vi "ManageAreaScanRoutines.vi"(0 "System no.":i32=1 min=1 step=1, 5 "error in (no error)":errorcluster) -> (19 "error out":errorcluster)   [LabVIEW 2020]
doc: "This VI allows to add or edit Area Scan Routines (FDR).\n\nRoutines can be managed on the controller directly or via text files."
uses:
  Message Cluster.ctl
  <vilib>/Utility/miscctls.llb/LVRowAndColumnTypeDef.ctl
panel:
  in  "Update from selected":bool
  in  "Calculate Velocity":bool
  in  "Mid. pos. step axis":dbl=0.1 format="%.4f"
  in  "Range step axis":dbl=0.1 format="%.4f"
  in  "Mid. pos. scan axis":dbl=0.1 format="%.4f"
  in  "Range scan axis":dbl=0.1 format="%.4f"
  in  "Name":string
  in  "Send to controller":bool
  in  "Board":i32 min=1 max=5 step=1
  in  "Threshold Level":dbl format="%.3f"
  in  "Centroid Method":i32
  in  "Target type":i32
  in  "Stop pos. option":i32
  in  "Velocity":dbl format="%.4f"
  in  "Frequency":dbl format="%.3f"
  in  "Max. rel. input level":dbl format="%.4f"
  in  "Min. rel. input level":dbl format="%.4f"
  in  "Step axis":string
  in  "Scan axis":string
  in  "stop":bool
  in  "Available Routines":string[][](table)
  # "Routine definition"
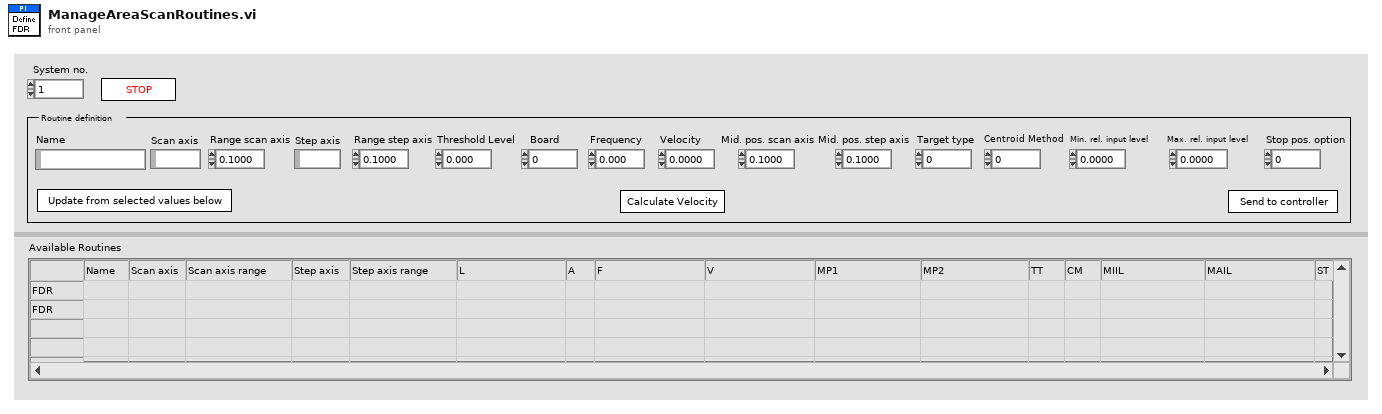
[diagram p1: front panel]
types:
  T1 = typedef "Message Cluster.ctl" = cluster{"Message":string, "Message Data":variant}
  T2 = typedef "LVRowAndColumnTypeDef.ctl" = cluster{"Row":i32, "Column":i32}
  T3 = cluster{"Scan axis":string, "Range scan axis":dbl, bool, "Mid. pos. scan axis":dbl}
  T4 = cluster{"Step axis":string, "Range step axis":dbl, bool, "Mid. pos. step axis":dbl}
  T5 = enum32{"Bad", "Idle", "Run top level", "Running"}
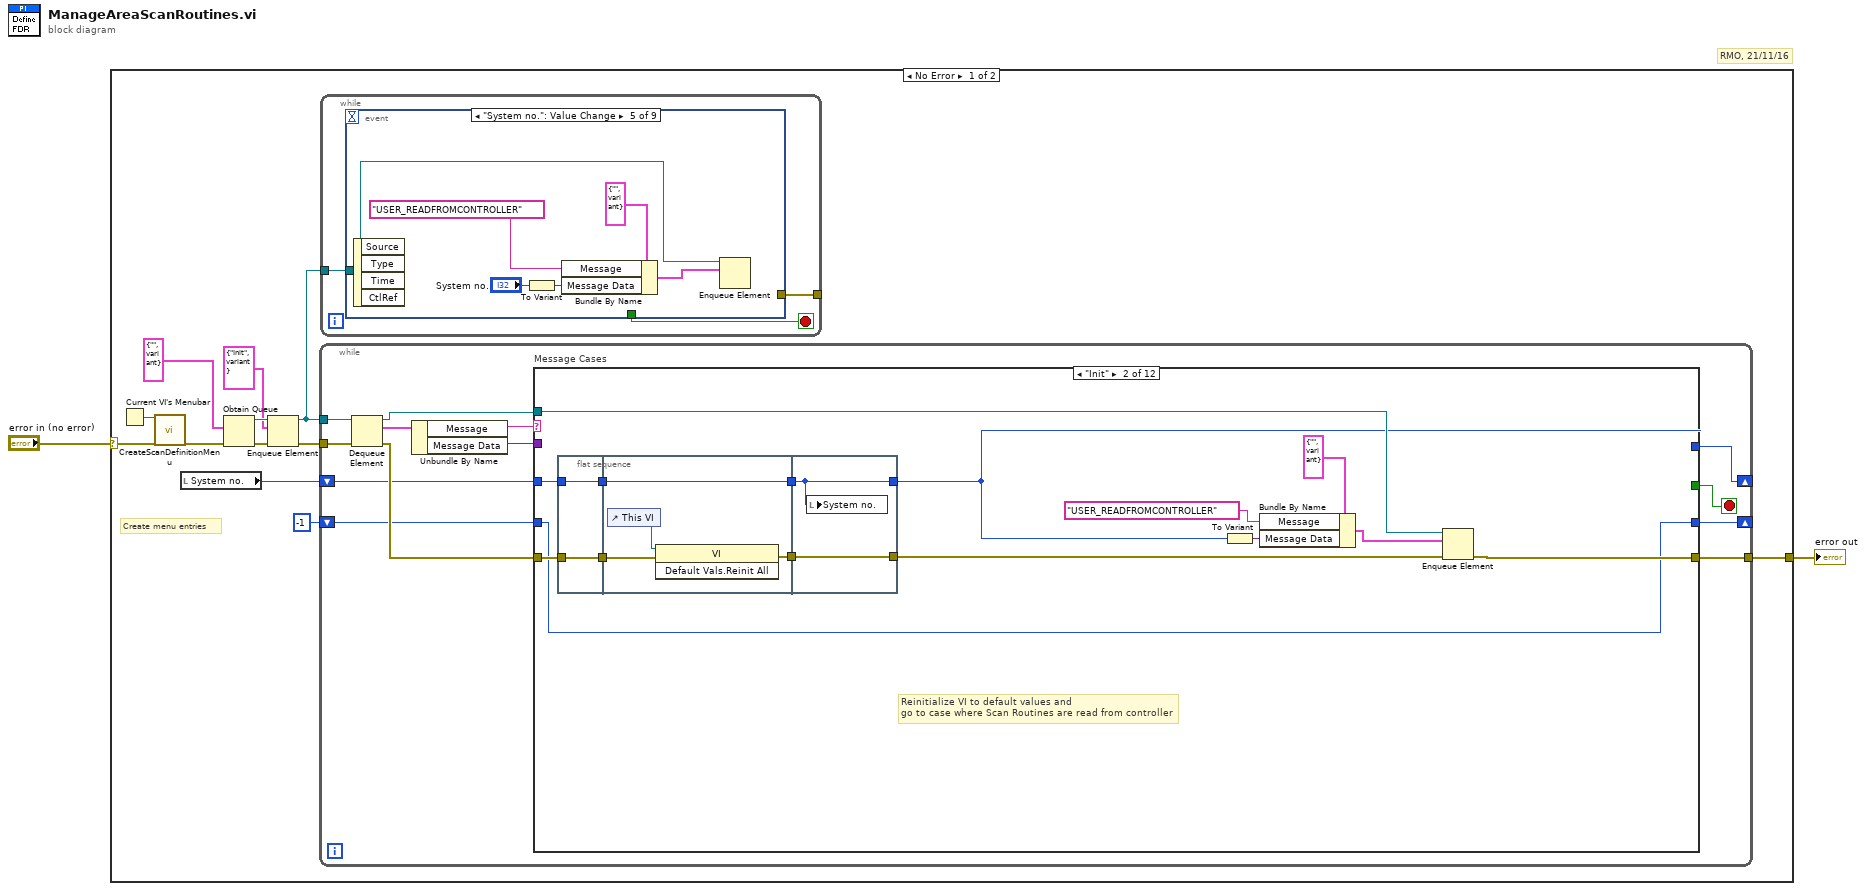
[diagram p0: block diagram]
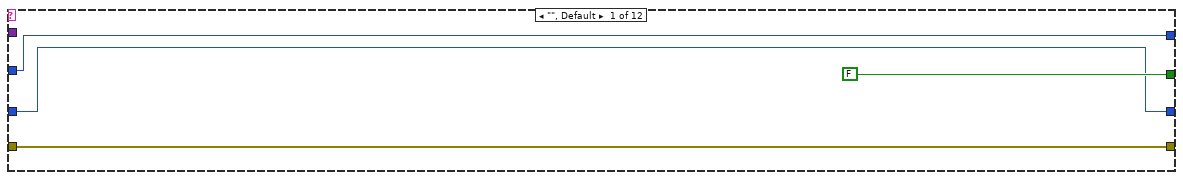
[diagram p2: hidden frame]
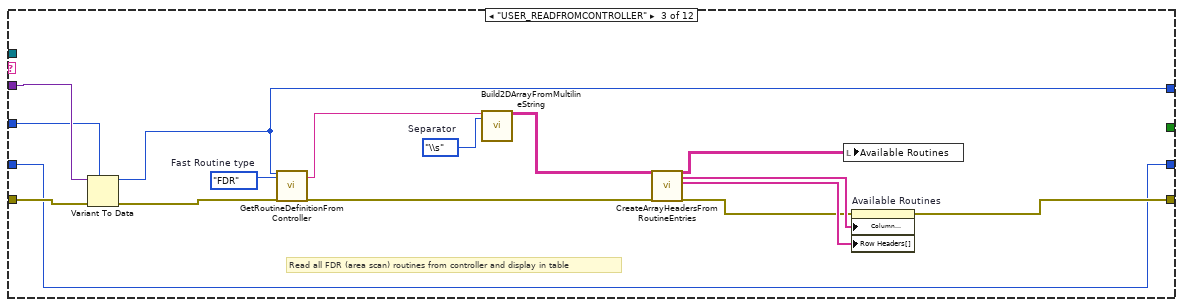
[diagram p3: hidden frame]
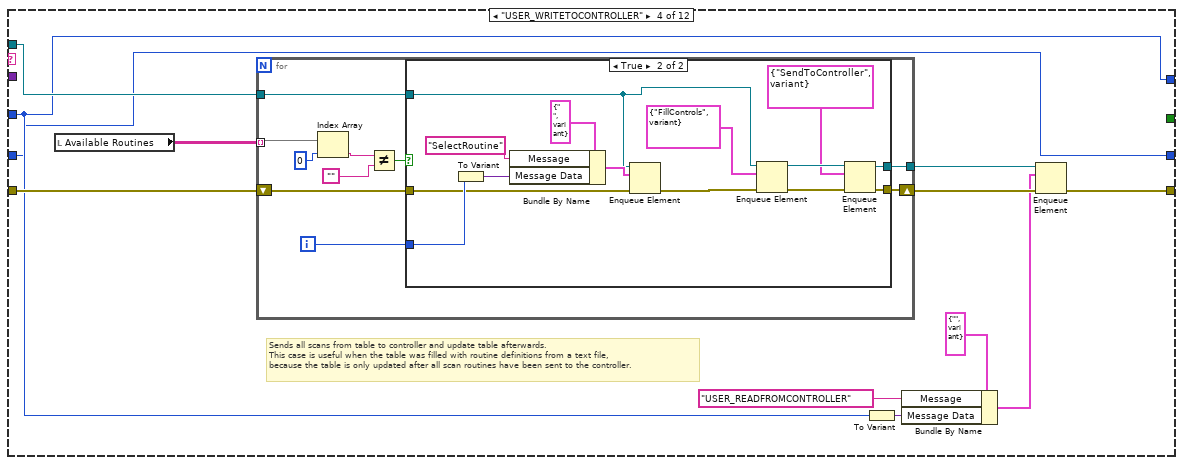
[diagram p4: hidden frame]
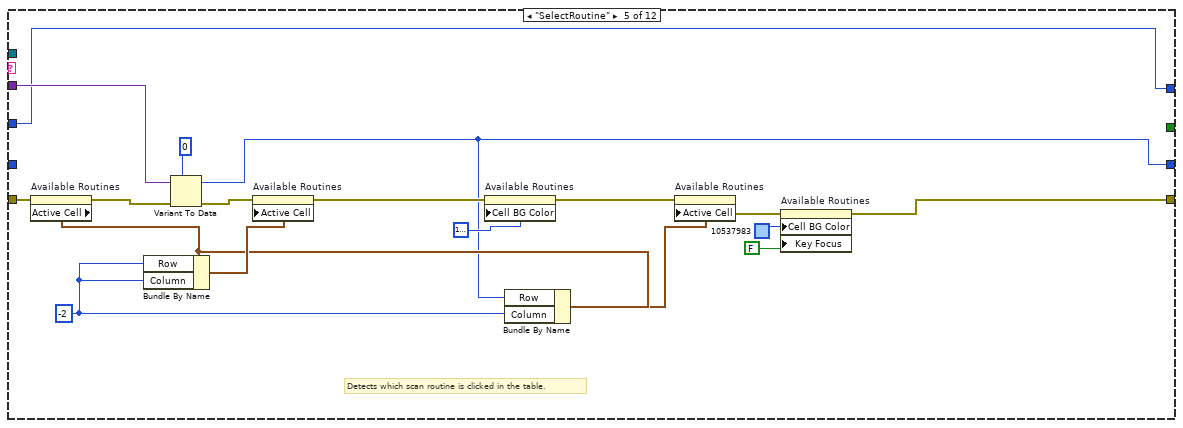
[diagram p6: hidden frame]
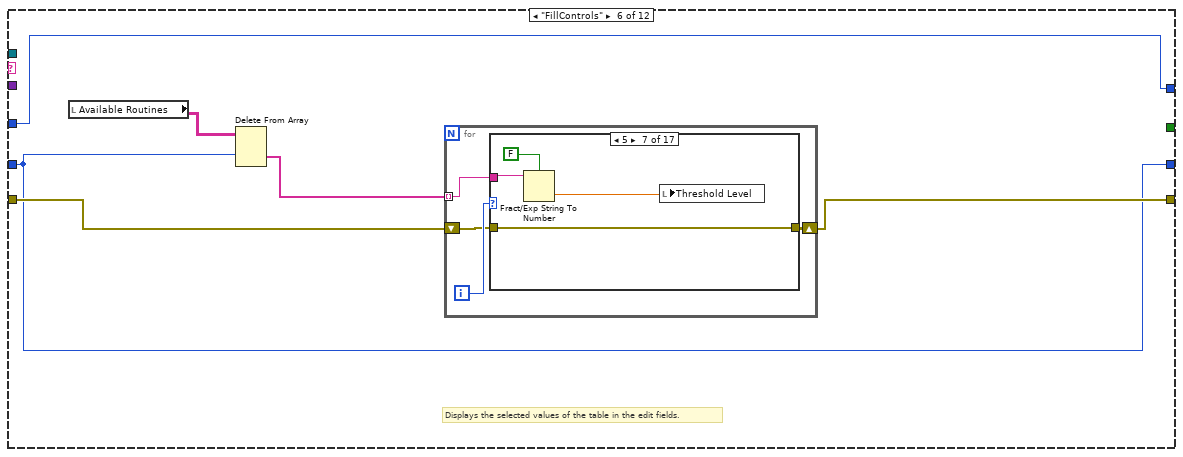
[diagram p7: hidden frame]
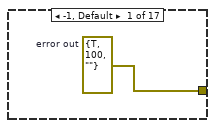
[diagram p8: hidden frame]
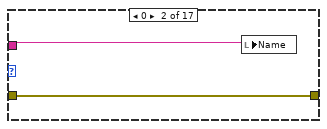
[diagram p9: hidden frame]
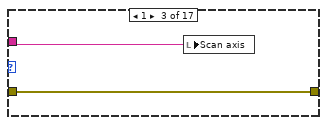
[diagram p10: hidden frame]
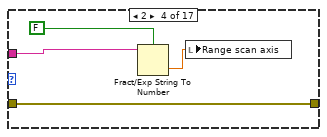
[diagram p11: hidden frame]
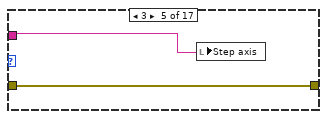
[diagram p12: hidden frame]
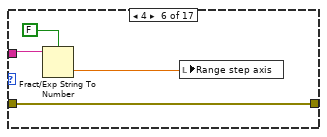
[diagram p13: hidden frame]
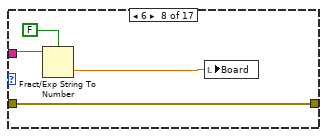
[diagram p14: hidden frame]
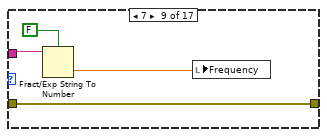
[diagram p15: hidden frame]
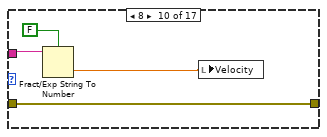
[diagram p16: hidden frame]
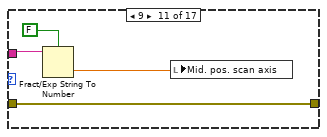
[diagram p17: hidden frame]
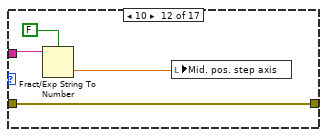
[diagram p18: hidden frame]
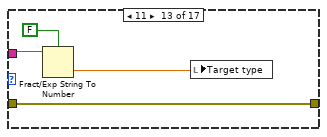
[diagram p19: hidden frame]
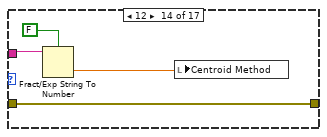
[diagram p20: hidden frame]
diagram:
  # "RMO, 21/11/16"
  n1 = case shown="No Error" "error in (no error)" {
    selector: "error in (no error)" -> [w5 w409]
    tunnel: [w6 w409] -> w2
    frame No Error {
      # "Create menu entries"
      n2 = Current VI's Menubar() -> (w14:refnum<k9>)
      n3 = call "CreateScanDefinitionMenu.vi"("menu reference"=w14, "error in (no error)"=w5) -> ("error out"=w8:errorcluster)  [unwired: 17 out]
      n4 = local read "System no."() -> (w3:i32)
      n5 = Obtain Queue(element data type=T1 {"Message"="", "Message Data"=variant} ("Message Cluster"), error in (no error)=w8) -> (queue out=w11:refnum<queue>, error out=w12:errorcluster)  [unwired: 2 in, 2 out]
      n6 = Enqueue Element(queue=w11, element=T1 {"Message"="Init", "Message Data"=variant}, error in (no error)=w12) -> (queue out=w7:refnum<queue>, error out=w9:errorcluster)  [unwired: 2 out]
      n7 = while {
        tunnel: w9 -> [w27]
        tunnel: w7 -> [w26]
        tunnel: [w21] -> w6
        shift-right: [w17] -> _
        shift-left: w3 -> [w20]
        shift-right: [w16] -> _
        shift-left: -1 ("Horizontal") -> [w15]
        stop <- w22 stop-if-true
        n8 = Dequeue Element(queue=w26, error in (no error)=w27) -> (queue out=w18:refnum<queue>, element=w25:T1, error out=w24:errorcluster)  [unwired: 2 out]
        n9 = Unbundle By Name(w25) -> ("Message"=w23:string, "Message Data"=w19:variant)
        n10 = case "Message Cases" shown="\"Init\"" w23 {
          tunnel: w24 -> [w31 w44 w61 w80 w124 w128 w203 w247 w284 w304 w331 w350]
          tunnel: [w31 w45 w64 w78 w110 w130 w202 w246 w281 w289 w333 w340] -> w21
          tunnel: [FALSE _ _ _ _ _ _ _ _ _ _ TRUE] -> w22
          tunnel: w20 -> [w29 w36 w58 w72 w111 w129 w197 w242 w280 w300 w329 w347]
          tunnel: w19 -> [_ _ w59 _ w126 _ _ _ _ _ _ _]
          tunnel: w18 -> [_ w46 _ w81 _ _ w201 _ _ _ _ _]
          tunnel: [w29 w32 w57 w72 w111 w129 w197 w242 w280 w300 w329 w347] -> w17
          tunnel: [w28 w38 w55 w71 w109 w127 w196 w241 w279 w286 w327 w339] -> w16
          tunnel: w15 -> [w28 w38 w55 w71 _ w127 w196 w241 w279 w286 w327 w339]
          frame "", Default {
          }
          frame "Init" {
            # "Reinitialize VI to default values and\ngo to case where Scan Routines are read from controller"
            n11 = flat-sequence {
              tunnel: w44 -> [w48]
              tunnel: [w48] -> w37
              tunnel: w36 -> [w47]
              tunnel: [w47] -> w35
              tunnel: w37 -> [w51]
              tunnel: w35 -> [w49]
              tunnel: [w50] -> w34
              tunnel: [w49] -> w33
              tunnel: [w54] -> w43
              tunnel: w34 -> [w54]
              tunnel: w33 -> [w53]
              tunnel: [w53] -> w32
              frame #0 {
              }
              frame #1 {
                n12 = control-ref of="This VI"() -> (w52:refnum<vi>)
                n13 = invoke class="VI" method="Default Vals.Reinit All"(reference=w52, error in=w51) -> (error out=w50:errorcluster)  [unwired: 1 in, 2 out]
              }
              frame #2 {
                n14 = local write "System no."(w53) -> ()
              }
            }
            n15 = To Variant(anything=w32) -> (Variant=w42:variant)
            n16 = Bundle By Name(cluster=T1 {"Message"="", "Message Data"=variant} ("Message Cluster"), "Message"="USER_READFROMCONTROLLER", "Message Data"=w42) -> (w40:T1)
            n17 = Enqueue Element(queue=w46, element=w40, error in (no error)=w43) -> (error out=w45:errorcluster)  [unwired: 3 out]
          }
          frame "USER_READFROMCONTROLLER" {
            w69 = enum16{"\\s", "\\t"}."\\s"  # Separator
            w70 = enum16{"FDG", "FDR"}."FDR"  # Fast Routine type
            # "Read all FDR (area scan) routines from controller and display in table"
            n18 = Variant To Data(error in=w61, type=w58, Variant=w59) -> (data=w57:i32, error out=w60:errorcluster)
            n19 = call "GetRoutineDefinitionFromController.vi"("System no."=w57, "Fast Routine type"=w70, "error in"=w60) -> ("Routine Definitons"=w56:string, "error out"=w63:errorcluster)  [unwired: 15 out]
            n20 = call "Build2DArrayFromMultilineString.vi"("String"=w56, "Separator"=w69) -> ("2D Array out"=w68:string[][])  [unwired: 17 out]
            n21 = call "CreateArrayHeadersFromRoutineEntries.vi"("Available Routines"=w68, "error in"=w63) -> ("Available Routines out"=w67:string[][], "Column Headers"=w66:string[], "Row Headers"=w65:string[], "error out"=w62:errorcluster)  [unwired: 14 out]
            n22 = local write "Available Routines"(w67) -> ()
            n23 = property on="Available Routines" class="Tbl (strict)"(error in=w62, "Column Headers[]"=w66, "Row Headers[]"=w65) -> (error out=w64:errorcluster)  [unwired: 1 in, 1 out]
          }
          frame "USER_WRITETOCONTROLLER" {
            # "Sends all scans from table to controller and update table afterwards.\nThis case is useful when the table was filled with routine definitions from a text file,\nbecause the table is only updated after all scan routines have been sent to the controller."
            n24 = local read "Available Routines"() -> (w82:string[][])
            n25 = for {
              tunnel: w82 -> [w88] mode=indexing
              tunnel: w81 -> [w91]
              shift-right: [w89] -> w79
              shift-left: w80 -> [w90]
              tunnel: [w83] -> w77
              i -> [w92]
              n26 = Index Array(array=w88, index=0) -> (element=w86:string)
              n27 = Not Equal?(x=w86, y="") -> (x != y?=w84:bool)
              n28 = case shown="True" w84 {
                tunnel: w92 -> [_ w105]
                tunnel: w91 -> [w93 w96]
                tunnel: w90 -> [w94 w99]
                tunnel: [w94 w101] -> w89
                tunnel: [w93 w100] -> w83
                frame False {
                }
                frame True {
                  n29 = To Variant(anything=w105) -> (Variant=w106:variant)
                  n30 = Bundle By Name(cluster=T1 {"Message"="  ", "Message Data"=variant} ("Message Cluster"), "Message"="SelectRoutine", "Message Data"=w106) -> (w97:T1)
                  n31 = Enqueue Element(queue=w96, element=w97, error in (no error)=w99) -> (error out=w98:errorcluster)  [unwired: 3 out]
                  n32 = Enqueue Element(queue=w96, element=T1 {"Message"="FillControls", "Message Data"=variant}, error in (no error)=w98) -> (queue out=w103:refnum<queue>, error out=w104:errorcluster)  [unwired: 2 out]
                  n33 = Enqueue Element(queue=w103, element=T1 {"Message"="SendToController", "Message Data"=variant}, error in (no error)=w104) -> (queue out=w100:refnum<queue>, error out=w101:errorcluster)  [unwired: 2 out]
                }
              }
            }
            n34 = To Variant(anything=w72) -> (Variant=w76:variant)
            n35 = Bundle By Name(cluster=T1 {"Message"="", "Message Data"=variant} ("Message Cluster"), "Message"="USER_READFROMCONTROLLER", "Message Data"=w76) -> (w74:T1)
            n36 = Enqueue Element(queue=w77, element=w74, error in (no error)=w79) -> (error out=w78:errorcluster)  [unwired: 3 out]
          }
          frame "SelectRoutine" {
            w116 = -2 ("Row")
            # "Detects which scan routine is clicked in the table."
            n37 = property on="Available Routines" class="Tbl (strict)"(error in=w124) -> (error out=w112:errorcluster, "Active Cell"=w117:T2)  [unwired: 1 in, 1 out]
            n38 = Bundle By Name(cluster=w117, "Row"=w116, "Column"=w116) -> (w121:T2)
            n39 = Variant To Data(error in=w112, type=0 ("Horizontal"), Variant=w126) -> (data=w109:i32, error out=w123:errorcluster)
            n40 = property on="Available Routines" class="Tbl (strict)"(error in=w123, "Active Cell"=w121) -> (error out=w122:errorcluster)  [unwired: 1 in, 1 out]
            n41 = property on="Available Routines" class="Tbl (strict)"(error in=w122, "Cell BG Color"=u32 16777225 ("Color Box")) -> (error out=w120:errorcluster)  [unwired: 1 in, 1 out]
            n42 = Bundle By Name(cluster=w117, "Row"=w109, "Column"=w116) -> (w115:T2)
            n43 = property on="Available Routines" class="Tbl (strict)"(error in=w120, "Active Cell"=w115) -> (error out=w119:errorcluster)  [unwired: 1 in, 1 out]
            n44 = property on="Available Routines" class="Tbl (strict)"(error in=w119, "Cell BG Color"=u32 10537983 ("Color Box"), "Key Focus"=FALSE) -> (error out=w110:errorcluster)  [unwired: 1 in, 1 out]
          }
          frame "FillControls" {
            # "Displays the selected values of the table in the edit fields."
            n45 = local read "Available Routines"() -> (w132:string[][])
            n46 = Delete From Array(array=w132, index (row)=w127) -> (deleted portion=w131:string[])  [unwired: 2 in, 1 out]
            n47 = for {
              tunnel: w131 -> [w136] mode=indexing
              shift-right: [w133] -> w130
              shift-left: w128 -> [w134]
              i -> [w135]
              n48 = case shown="5" w135 {
                tunnel: w136 -> [_ w138 w141 w143 w146 w150 w154 w158 w162 w166 w170 w174 w178 w182 w186 w190 w194]
                tunnel: w134 -> [_ w139 w140 w145 w147 w151 w155 w159 w163 w167 w171 w175 w179 w183 w187 w191 w195]
                tunnel: [w137 w139 w140 w145 w147 w151 w155 w159 w163 w167 w171 w175 w179 w183 w187 w191 w195] -> w133
                frame -1, Default {
                  w137 = errorcluster {"status"=TRUE, "code"=100, "source"=""}  # error out
                }
                frame 0 {
                  n49 = local write "Name"(w138) -> ()
                }
                frame 1 {
                  n50 = local write "Scan axis"(w141) -> ()
                }
                frame 2 {
                  n51 = Fract/Exp String To Number(use system decimal point (T)=FALSE, string=w143) -> (number=w142:dbl)  [unwired: 3 out]
                  n52 = local write "Range scan axis"(w142) -> ()
                }
                frame 3 {
                  n53 = local write "Step axis"(w146) -> ()
                }
                frame 4 {
                  n54 = Fract/Exp String To Number(use system decimal point (T)=FALSE, string=w150) -> (number=w149:dbl)  [unwired: 3 out]
                  n55 = local write "Range step axis"(w149) -> ()
                }
                frame 5 {
                  n56 = Fract/Exp String To Number(use system decimal point (T)=FALSE, string=w154) -> (number=w153:dbl)  [unwired: 3 out]
                  n57 = local write "Threshold Level"(w153) -> ()
                }
                frame 6 {
                  n58 = Fract/Exp String To Number(use system decimal point (T)=FALSE, string=w158) -> (number=w157:dbl)  [unwired: 3 out]
                  n59 = local write "Board"(w157) -> ()
                }
                frame 7 {
                  n60 = Fract/Exp String To Number(use system decimal point (T)=FALSE, string=w162) -> (number=w161:dbl)  [unwired: 3 out]
                  n61 = local write "Frequency"(w161) -> ()
                }
                frame 8 {
                  n62 = Fract/Exp String To Number(use system decimal point (T)=FALSE, string=w166) -> (number=w165:dbl)  [unwired: 3 out]
                  n63 = local write "Velocity"(w165) -> ()
                }
                frame 9 {
                  n64 = Fract/Exp String To Number(use system decimal point (T)=FALSE, string=w170) -> (number=w169:dbl)  [unwired: 3 out]
                  n65 = local write "Mid. pos. scan axis"(w169) -> ()
                }
                frame 10 {
                  n66 = Fract/Exp String To Number(use system decimal point (T)=FALSE, string=w174) -> (number=w173:dbl)  [unwired: 3 out]
                  n67 = local write "Mid. pos. step axis"(w173) -> ()
                }
                frame 11 {
                  n68 = Fract/Exp String To Number(use system decimal point (T)=FALSE, string=w178) -> (number=w177:dbl)  [unwired: 3 out]
                  n69 = local write "Target type"(w177) -> ()
                }
                frame 12 {
                  n70 = Fract/Exp String To Number(use system decimal point (T)=FALSE, string=w182) -> (number=w181:dbl)  [unwired: 3 out]
                  n71 = local write "Centroid Method"(w181) -> ()
                }
                frame 13 {
                  n72 = Fract/Exp String To Number(use system decimal point (T)=FALSE, string=w186) -> (number=w185:dbl)  [unwired: 3 out]
                  n73 = local write "Min. rel. input level"(w185) -> ()
                }
                frame 14 {
                  n74 = Fract/Exp String To Number(use system decimal point (T)=FALSE, string=w190) -> (number=w189:dbl)  [unwired: 3 out]
                  n75 = local write "Max. rel. input level"(w189) -> ()
                }
                frame 15 {
                  n76 = Fract/Exp String To Number(use system decimal point (T)=FALSE, string=w194) -> (number=w193:dbl)  [unwired: 3 out]
                  n77 = local write "Stop pos. option"(w193) -> ()
                }
              }
            }
          }
          frame "SendToControllerAndUpdate" {
            # "When pressing Return button or \"Send to controller\" button, Scan is defined on controller and USER_READFROMCONTROLLER case is triggered"
            n78 = Not Equal?(x="Name", y="") -> (x != y?=w198:bool)
            n79 = case shown="True" w198 {
              tunnel: w203 -> [w204 w221]
              tunnel: w197 -> [_ w205]
              tunnel: [w204 w240] -> w202
              tunnel: w201 -> [_ w239]
              tunnel: "Name" -> [_ w210]
              frame False {
              }
              frame True {
                w214 = TRUE
                w232 = TRUE
                n80 = Bundle(w214, "Frequency"="Frequency") -> (w219:cluster{bool, "Frequency":dbl})  [unwired: 1 out]
                n81 = Bundle(w214, "Stop pos. option"="Stop pos. option") -> (w217:cluster{bool, "Stop pos. option":i32})  [unwired: 1 out]
                n82 = Bundle(w214, "Min. rel. input level"="Min. rel. input level") -> (w215:cluster{bool, "Min. rel. input level":dbl})  [unwired: 1 out]
                n83 = Bundle(w214, "Max. rel. input level"="Max. rel. input level") -> (w212:cluster{bool, "Max. rel. input level":dbl})  [unwired: 1 out]
                n84 = Bundle("Scan axis"="Scan axis", "Range scan axis"="Range scan axis", w214, "Mid. pos. scan axis"="Mid. pos. scan axis") -> (w229:T3)  [unwired: 1 out]
                n85 = Bundle("Step axis"="Step axis", "Range step axis"="Range step axis", w214, "Mid. pos. step axis"="Mid. pos. step axis") -> (w222:T4)  [unwired: 1 out]
                n86 = Bundle(w232, "Centroid Method"="Centroid Method") -> (w231:cluster{bool, "Centroid Method":i32})  [unwired: 1 out]
                n87 = Bundle(w232, "Target type"="Target type") -> (w234:cluster{bool, "Target type":i32})  [unwired: 1 out]
                n88 = Bundle(w232, "Velocity"="Velocity") -> (w236:cluster{bool, "Velocity":dbl})  [unwired: 1 out]
                n89 = call "FDR.vi"("System no."=w205, "Board"="Board", "Routinename"=w210, "Scan axis settings"=w229, "Step axis settings"=w222, "error in"=w221, "Threshold level"="Threshold Level", "Frequency settings"=w219, "Velocity settings"=w236, "Stop position option settings"=w217, "Target type settings"=w234, "Min. relative input level (MIIL) settings"=w215, "Centroid method settings"=w231, "Max. relative input level (MAIL) settings"=w212) -> ("error out"=w211:errorcluster)  [unwired: 5 out]
                n90 = To Variant(anything=w205) -> (Variant=w209:variant)
                n91 = Bundle By Name(cluster=T1 {"Message"="", "Message Data"=variant} ("Message Cluster"), "Message"="USER_READFROMCONTROLLER", "Message Data"=w209) -> (w206:T1)
                n92 = Enqueue Element(queue=w239, element=w206, error in (no error)=w211) -> (error out=w240:errorcluster)  [unwired: 3 out]
              }
            }
          }
          frame "SendToController" {
            # "Defines area scan routine on controller."
            n93 = local read "Name"() -> (w244:string)
            n94 = Not Equal?(x=w244, y="") -> (x != y?=w245:bool)
            n95 = case shown="True" w245 {
              tunnel: w247 -> [w248 w267]
              tunnel: w242 -> [_ w262]
              tunnel: w244 -> [_ w249]
              tunnel: [w248 w250] -> w246
              frame False {
              }
              frame True {
                w269 = TRUE
                w276 = TRUE
                n96 = local read "Max. rel. input level"() -> (w251:dbl)
                n97 = local read "Min. rel. input level"() -> (w252:dbl)
                n98 = local read "Mid. pos. scan axis"() -> (w258:dbl)
                n99 = local read "Mid. pos. step axis"() -> (w255:dbl)
                n100 = local read "Centroid Method"() -> (w266:i32)
                n101 = local read "Stop pos. option"() -> (w253:i32)
                n102 = local read "Threshold Level"() -> (w263:dbl)
                n103 = local read "Range scan axis"() -> (w259:dbl)
                n104 = local read "Range step axis"() -> (w256:dbl)
                n105 = local read "Target type"() -> (w265:i32)
                n106 = local read "Frequency"() -> (w254:dbl)
                n107 = local read "Scan axis"() -> (w260:string)
                n108 = local read "Step axis"() -> (w257:string)
                n109 = local read "Velocity"() -> (w264:dbl)
                n110 = local read "Board"() -> (w261:i32)
                n111 = Bundle(w269, "Frequency"=w254) -> (w272:cluster{bool, "Frequency":dbl})  [unwired: 1 out]
                n112 = Bundle(w269, "Stop pos. option"=w253) -> (w271:cluster{bool, "Stop pos. option":i32})  [unwired: 1 out]
                n113 = Bundle(w269, "Min. rel. input level"=w252) -> (w270:cluster{bool, "Min. rel. input level":dbl})  [unwired: 1 out]
                n114 = Bundle(w269, "Max. rel. input level"=w251) -> (w268:cluster{bool, "Max. rel. input level":dbl})  [unwired: 1 out]
                n115 = Bundle("Scan axis"=w260, "Range scan axis"=w259, w269, "Mid. pos. scan axis"=w258) -> (w274:T3)  [unwired: 1 out]
                n116 = Bundle("Step axis"=w257, "Range step axis"=w256, w269, "Mid. pos. step axis"=w255) -> (w273:T4)  [unwired: 1 out]
                n117 = Bundle(w276, "Centroid Method"=w266) -> (w275:cluster{bool, "Centroid Method":i32})  [unwired: 1 out]
                n118 = Bundle(w276, "Target type"=w265) -> (w277:cluster{bool, "Target type":i32})  [unwired: 1 out]
                n119 = Bundle(w276, "Velocity"=w264) -> (w278:cluster{bool, "Velocity":dbl})  [unwired: 1 out]
                n120 = call "FDR.vi"("System no."=w262, "Board"=w261, "Routinename"=w249, "Scan axis settings"=w274, "Step axis settings"=w273, "error in"=w267, "Threshold level"=w263, "Frequency settings"=w272, "Velocity settings"=w278, "Stop position option settings"=w271, "Target type settings"=w277, "Min. relative input level (MIIL) settings"=w270, "Centroid method settings"=w275, "Max. relative input level (MAIL) settings"=w268) -> ("error out"=w250:errorcluster)  [unwired: 5 out]
              }
            }
          }
          frame "USER_SAVETOFILE" {
            w285 = enum16{"FDG", "FDR"}."FDR"  # Fast Routine type
            # "Saves all FDR routines to text file."
            n121 = call "GetRoutineDefinitionFromController.vi"("System no."=w280, "Fast Routine type"=w285, "error in"=w284) -> ("Routine Definitons"=w282:string, "error out"=w283:errorcluster)  [unwired: 15 out]
            n122 = Write to Text File(text=w282, error in=w283) -> (error out=w281:errorcluster)  [unwired: 4 out]
          }
          frame "OpenCalculator" {
            # "Open calculator window."
            n123 = vi-ref "CalculateAreaScanVelocity.vi"() -> (w301:refnum<vi>)
            n124 = property class="VI"(reference=w301, error in=w304) -> (error out=w303:errorcluster, "Exec.State"=w306:T5)  [unwired: 1 out]
            n125 = case shown="\"Bad\", Default" w306 {
              tunnel: w303 -> [w319 w321 w323 w325]
              tunnel: [TRUE TRUE FALSE ("Wait Until Done") FALSE ("Wait Until Done")] -> w305
              tunnel: [w319 w321 w323 w325] -> w302
              frame "Bad", Default {
              }
              frame "Idle" {
              }
              frame "Run top level" {
              }
              frame "Running" {
              }
            }
            n126 = case shown="False" w305 {
              tunnel: w301 -> [w309 w316]
              tunnel: w302 -> [w310 w315]
              tunnel: [w308 w312] -> w298
              tunnel: [w307 w311] -> w299
              frame False {
                n127 = invoke class="VI" method="FP.Open"(reference=w309, error in=w310) -> (reference out=w307:refnum<vi>, error out=w308:errorcluster)  [unwired: 3 in, 3 out]
              }
              frame True {
                n128 = invoke class="VI" method="Run VI"(reference=w316, error in=w315, "Wait until done"=FALSE ("Wait Until Done"), "Auto Dispose Ref"=TRUE ("Auto Dispose Reference")) -> (reference out=w313:refnum<vi>, error out=w314:errorcluster)  [unwired: 1 in, 3 out]
                n129 = invoke class="VI" method="FP.Open"(reference=w313, error in=w314) -> (reference out=w311:refnum<vi>, error out=w312:errorcluster)  [unwired: 3 in, 3 out]
              }
            }
            n130 = local read "Target type"() -> (w292:i32)
            n131 = invoke class="VI" method="Ctrl Val.Set"(reference=w299, error in=w298, "Control Name"="Target type", "Value"=w292) -> (reference out=w297:refnum<vi>, error out=w296:errorcluster)  [unwired: 1 in, 3 out]
            n132 = local read "Frequency"() -> (w293:dbl)
            n133 = invoke class="VI" method="Ctrl Val.Set"(reference=w297, error in=w296, "Control Name"="Frequency", "Value"=w293) -> (reference out=w291:refnum<vi>, error out=w290:errorcluster)  [unwired: 1 in, 3 out]
            n134 = invoke class="VI" method="Ctrl Val.Set"(reference=w291, error in=w290, "Control Name"="Calculate", "Value"=TRUE) -> (error out=w289:errorcluster)  [unwired: 1 in, 4 out]
          }
          frame "USER_LOADFROMFILE" {
            w338 = enum16{"\\s", "\\t"}."\\s"  # Separator
            # "Load all area scan routines from text file and display in table"
            n135 = Read from Text File(error in=w331) -> (text=w328:string, error out=w330:errorcluster)  [unwired: 5 out]
            n136 = call "Build2DArrayFromMultilineString.vi"("String"=w328, "Separator"=w338) -> ("2D Array out"=w337:string[][])  [unwired: 17 out]
            n137 = call "CreateArrayHeadersFromRoutineEntries.vi"("Available Routines"=w337, "error in"=w330) -> ("Available Routines out"=w336:string[][], "Column Headers"=w335:string[], "Row Headers"=w334:string[], "error out"=w332:errorcluster)  [unwired: 14 out]
            n138 = local write "Available Routines"(w336) -> ()
            n139 = property on="Available Routines" class="Tbl (strict)"(error in=w332, "Column Headers[]"=w335, "Row Headers[]"=w334) -> (error out=w333:errorcluster)  [unwired: 1 in, 1 out]
          }
          frame "Exit" {
            w348 = T2 {"Row"=0, "Column"=0} ("Selection Start")
            # "Close calculator window before stopping this VI."
            n140 = property on="Available Routines" class="Tbl (strict)"(error in=w350, "Selection Start"=w348, "Selection Size"=w348) -> (error out=w349:errorcluster)  [unwired: 1 in, 1 out]
            n141 = property on="Available Routines" class="Tbl (strict)"(error in=w349, "Cell BG Color"=u32 16777225 ("Color Box")) -> (error out=w344:errorcluster)  [unwired: 1 in, 1 out]
            n142 = vi-ref "CalculateAreaScanVelocity.vi"() -> (w342:refnum<vi>)
            n143 = property class="VI"(reference=w342, error in=w344) -> (error out=w345:errorcluster, "Exec.State"=w346:T5)  [unwired: 1 out]
            n144 = case shown="\"Running\"" w346 {
              tunnel: w345 -> [w359 w361 w363 w365]
              tunnel: [FALSE FALSE TRUE ("Wait Until Done") TRUE ("Wait Until Done")] -> w343
              tunnel: [w359 w361 w363 w365] -> w341
              frame "Bad", Default {
              }
              frame "Idle" {
              }
              frame "Run top level" {
              }
              frame "Running" {
              }
            }
            n145 = case shown="True" w343 {
              tunnel: w342 -> [_ w358]
              tunnel: w341 -> [w353 w355]
              tunnel: [w353 w354] -> w340
              frame False {
              }
              frame True {
                n146 = invoke class="VI" method="Abort VI"(reference=w358, error in=w355) -> (reference out=w357:refnum<vi>, error out=w356:errorcluster)  [unwired: 1 in, 1 out]
                n147 = invoke class="VI" method="FP.Close"(reference=w357, error in=w356) -> (error out=w354:errorcluster)  [unwired: 1 in, 2 out]
              }
            }
          }
        }
      }
      n148 = while {
        tunnel: w7 -> [w369]
        tunnel: [w368] -> _
        stop <- w367 stop-if-true
        n149 = event shown="[4] \"System no.\": Value Change" {
          selector: _ -> [_ _ _ _ _ _ _ _ _]
          dyn-events: _ -> [_ _ _ _ _ _ _ _ _]
          timeout: _ -> [_ _ _ _ _ _ _ _ _]
          tunnel: w369 -> [_ w372 w377 w381 w390 w399 w402 w404 w406]
          tunnel: [_ w370 w375 w380 _ w398 w401 w403 w407] -> w368
          tunnel: [_ "stop" TRUE _ _ _ _ _ _] -> w367
          event Timeout {
            n150 = event-data() -> ()  [unwired: 3 out]
          }
          event "stop": Value Change {
            n151 = event-data() -> ()  [unwired: 5 out]
            n152 = Enqueue Element(queue=w372, element=T1 {"Message"="Exit", "Message Data"=variant}) -> (error out=w370:errorcluster)  [unwired: 1 in, 3 out]
          }
          event Panel Close? {
            n153 = event-data() -> ()  [unwired: 5 out]
            n154 = Enqueue Element(queue=w377, element=T1 {"Message"="Exit", "Message Data"=variant}) -> (error out=w375:errorcluster)  [unwired: 1 in, 3 out]
            n155 = event-data() -> ()  [unwired: 1 in, 2 out]
          }
          event Menu Selection (User) {
            n156 = event-data() -> ("ItemTag"=w383:string)  [unwired: 1 out]
            n157 = local read "System no."() -> (w378:i32)
            n158 = To Variant(anything=w378) -> (Variant=w379:variant)
            n159 = Bundle By Name(cluster=T1 {"Message"="", "Message Data"=variant} ("Message Cluster"), "Message"=w383, "Message Data"=w379) -> (w382:T1)
            n160 = Enqueue Element(queue=w381, element=w382) -> (error out=w380:errorcluster)  [unwired: 1 in, 3 out]
          }
          event "System no.": Value Change {
            n161 = event-data() -> ()  [unwired: 5 out]
            n162 = To Variant(anything="System no.") -> (Variant=w386:variant)
            n163 = Bundle By Name(cluster=T1 {"Message"="", "Message Data"=variant} ("Message Cluster"), "Message"="USER_READFROMCONTROLLER", "Message Data"=w386) -> (w387:T1)
            n164 = Enqueue Element(queue=w390, element=w387) -> ()  [unwired: 1 in, 4 out]
          }
          event "Available Routines": Mouse Down {
            n165 = event-data() -> ("CtlRef"=w393:refnum<vi>)  [unwired: 1 out]
            n166 = property class="Tbl (strict)"(reference=w393) -> ("Selection Start"=w392:T2)  [unwired: 1 in, 2 out]
            n167 = Unbundle By Name(w392) -> ("Row"=w391:i32)
            n168 = To Variant(anything=w391) -> (Variant=w395:variant)
            n169 = Bundle By Name(cluster=T1 {"Message"="  ", "Message Data"=variant} ("Message Cluster"), "Message"="SelectRoutine", "Message Data"=w395) -> (w394:T1)
            n170 = Enqueue Element(queue=w399, element=w394) -> (error out=w398:errorcluster)  [unwired: 1 in, 3 out]
          }
          event "Send to controller": Value Change; "Send to controller": Key Down {
            n171 = event-data() -> ()  [unwired: 5 out]
            n172 = Enqueue Element(queue=w402, element=T1 {"Message"="SendToControllerAndUpdate", "Message Data"=variant}) -> (error out=w401:errorcluster)  [unwired: 1 in, 3 out]
          }
          event "Calculate Velocity": Value Change {
            n173 = event-data() -> ()  [unwired: 2 out]
            n174 = Enqueue Element(queue=w404, element=T1 {"Message"="OpenCalculator", "Message Data"=variant}) -> (error out=w403:errorcluster)  [unwired: 1 in, 3 out]
          }
          event "Update from selected": Value Change {
            n175 = event-data() -> ()  [unwired: 2 out]
            n176 = Enqueue Element(queue=w406, element=T1 {"Message"="FillControls", "Message Data"=variant}) -> (error out=w407:errorcluster)  [unwired: 1 in, 3 out]
          }
        }
      }
    }
    frame Error {
    }
  }
  "error out" <- w2
